vi "U2000_USB_PM_Configure_Cal_Zero.vi"(6 "Zero Mode":enum16{"ONCE", "ON", "OFF"}(ring), 7 "Cal Mode":enum16{"ONCE", "OFF", "ON"}(ring), 8 "error in (no error)":errorcluster, 9 "Cal ALL [F]":bool, 11 "VISA resource name":refnum<visa-resource-name>) -> (0 "error out":errorcluster, 2 "Cal Status":bool, 3 "VISA resource name out":refnum<visa-resource-name>)   [LabVIEW 2015]
doc: "Performs a zeroing routine for both internal and external zeroing types."
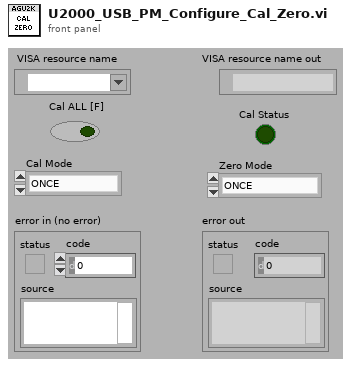
[diagram p1: front panel]
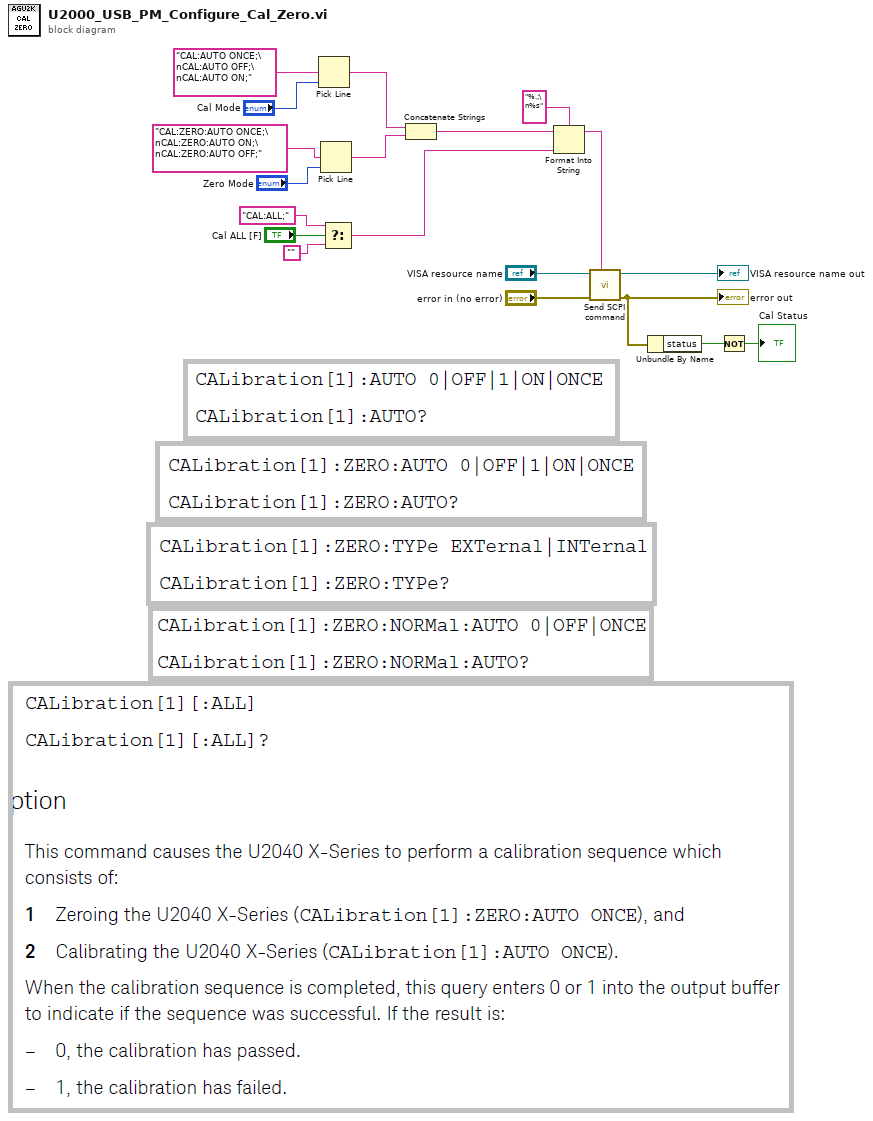
[diagram p0: block diagram]
diagram:
  n1 = Pick Line(multi-line string="CAL:AUTO ONCE;\nCAL:AUTO OFF;\nCAL:AUTO ON;" ("Zero Once"), line index="Cal Mode") -> (output string=w11:string)  [unwired: 1 in]
  n2 = Pick Line(multi-line string="CAL:ZERO:AUTO ONCE;\nCAL:ZERO:AUTO ON;\nCAL:ZERO:AUTO OFF;" ("Zero Once"), line index="Zero Mode") -> (output string=w10:string)  [unwired: 1 in]
  n3 = Select(t="CAL:ALL;", s="Cal ALL [F]", f="") -> (s? t:f=w6:string)
  n4 = Concatenate Strings(w11, w10) -> (w8:string)
  n5 = Format Into String(format string="%.;\n%s", initial string=w8, w6) -> (resulting string=w5:string)  [unwired: 1 in, 1 out]
  n6 = call "Send SCPI command.vi"("Send SCPI Command"=w5, "error in (no error)"="error in (no error)", "VISA resource name"="VISA resource name") -> ("error out"=w3:errorcluster, "VISA resource name out"=→"VISA resource name out":refnum<visa-resource-name>)  [unwired: 7 in]
  "error out" <- w3
  n7 = Unbundle By Name(w3) -> ("status"=w2:bool)
  n8 = Not(x=w2) -> (.not. x?=→"Cal Status":bool)
